vi "Mem_ObtainPTRQueue.vi"(8 "error in (no error)":errorcluster) -> (0 "error out":errorcluster, 3 "queue out":refnum<queue>)   [LabVIEW 2019, in "Memory Data Access.lvlib"]
uses:
  Memory Data Access.lvlib
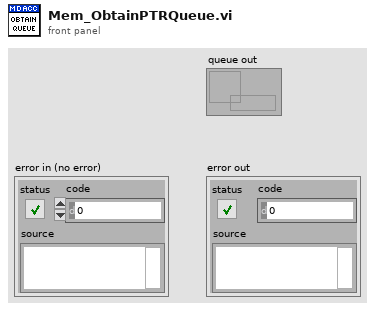
[diagram p1: front panel]
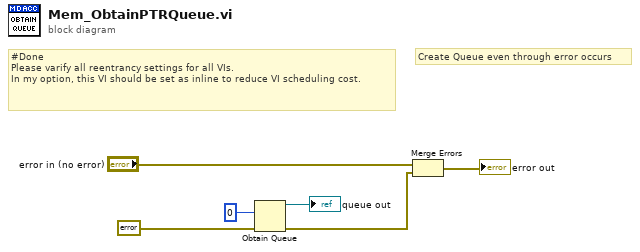
[diagram p0: block diagram]
diagram:
  # "Create Queue even through error occurs"
  # "#Done\nPlease varify all reentrancy settings for all VIs.\nIn my option, this VI should be set as inline to reduce VI scheduling cost."
  n1 = Obtain Queue(element data type=u64 0, error in (no error)=errorcluster {"status"=FALSE, "code"=0, "source"=""}) -> (queue out=→"queue out":refnum<queue>, error out=w2:errorcluster)  [unwired: 3 in, 1 out]
  n2 = Merge Errors("error in (no error)", w2) -> (→"error out":errorcluster)
